vi "First Order System Demo.vi"() -> ()   [LabVIEW 2021]
panel:
  in  "Stop Button":bool
  out "First Order System Step Response":waveform(dbl)[](graph)
  in  "Final Value":dbl=1.0
  in  "Initial Value":dbl
  in  "Time constant [s]":dbl(slide)=1.0 scale=0.0..10.0
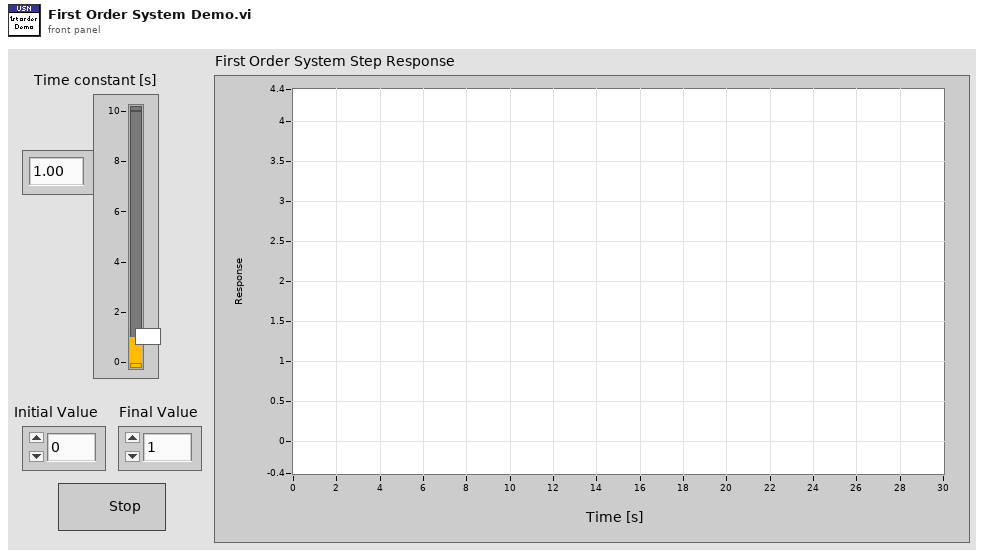
[diagram p1: front panel]
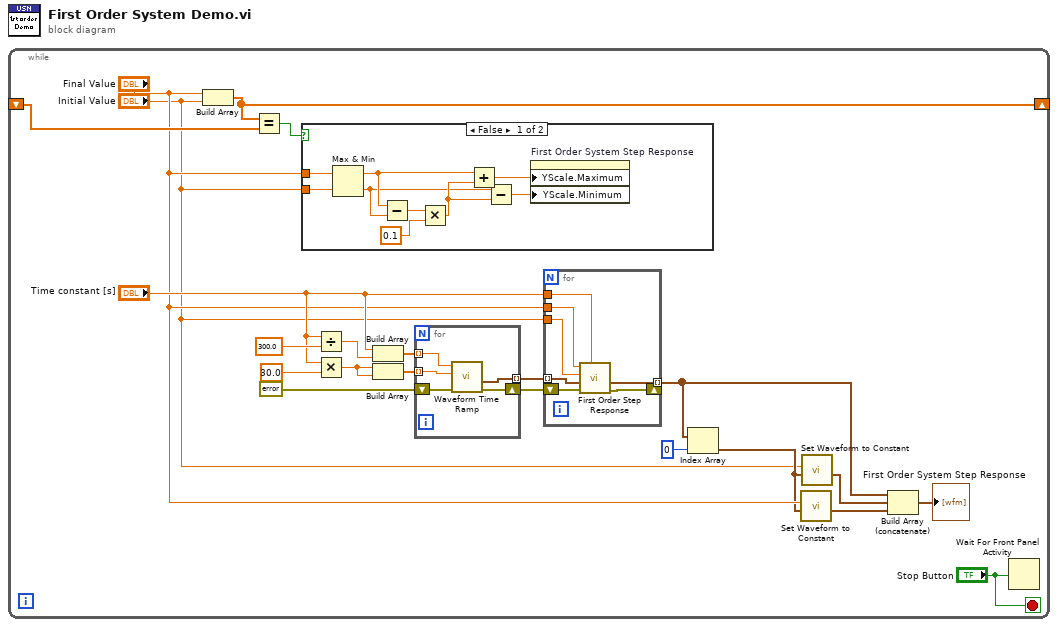
[diagram p0: block diagram]
diagram:
  n1 = while {
    shift-right: [w14] -> _
    shift-left: _ -> [w20]
    stop <- "Stop Button" stop-if-true
    n2 = Build Array("Final Value", "Initial Value") -> (w14:dbl[])
    n3 = Equal?(x=w14, y=w20) -> (x = y?=w19:bool)
    n4 = case shown="False" w19 {
      tunnel: "Final Value" -> [w29 _]
      tunnel: "Initial Value" -> [w28 _]
      frame False {
        n5 = Max & Min(x=w29, y=w28) -> (max(x,y)=w33:dbl, min(x,y)=w32:dbl)
        n6 = Subtract(x=w33, y=w32) -> (x-y=w36:dbl)
        n7 = Multiply(x=w36, y=0.1) -> (x*y=w34:dbl)
        n8 = Add(x=w33, y=w34) -> (x+y=w31:dbl)
        n9 = Subtract(x=w32, y=w34) -> (x-y=w30:dbl)
        n10 = property on="First Order System Step Response" class="WFGraph (strict)"("YScale.Maximum"=w31, "YScale.Minimum"=w30) -> ()  [unwired: 2 in, 2 out]
      }
      frame True {
      }
    }
    n11 = Divide(x="Time constant [s]", y=300.0) -> (x/y=w15:dbl)
    n12 = Multiply(x="Time constant [s]", y=30.0 ("x")) -> (x*y=w12:dbl)
    n13 = Build Array("Time constant [s]", w15) -> (w17:dbl[])
    n14 = Build Array(w12, w12) -> (w16:dbl[])
    n15 = for {
      tunnel: [w27] -> w11 mode=indexing
      tunnel: w17 -> [w26] mode=indexing
      tunnel: w16 -> [w25] mode=indexing
      shift-right: [w24] -> w2
      shift-left: errorcluster {"status"=FALSE, "code"=0, "source"=""} ("Error Out") -> [w23]
      n16 = call "Waveform Time Ramp.vi"("Error In"=w23, "End [s]"=w25, "dt [s]"=w26) -> ("Error Out"=w24:errorcluster, "Waveform Time Ramp"=w27:waveform(dbl))  [unwired: 7 in]
    }
    n17 = for {
      tunnel: "Initial Value" -> [w43]
      tunnel: "Final Value" -> [w42]
      tunnel: [w41] -> w9 mode=indexing
      tunnel: w11 -> [w39] mode=indexing
      tunnel: "Time constant [s]" -> [w40]
      shift-right: [w38] -> _
      shift-left: w2 -> [w37]
      n18 = call "First Order Step Response.vi"("Time constant [s]"=w40, "Error In"=w37, "Time Vector [s]"=w39, "Initial Value"=w43, "Final Value"=w42) -> ("Error Out"=w38:errorcluster, "Response"=w41:waveform(dbl))  [unwired: 5 in]
    }
    n19 = Index Array(array=w9, index=0) -> (element=w5:waveform(dbl))
    n20 = call "Set Waveform to Constant.vi"("Original Waveform"=w5, "New Value"="Final Value") -> ("New Waveform"=w7:waveform(dbl))  [unwired: 8 in, 1 out]
    n21 = call "Set Waveform to Constant.vi"("Original Waveform"=w5, "New Value"="Initial Value") -> ("New Waveform"=w3:waveform(dbl))  [unwired: 8 in, 1 out]
    n22 = Build Array (concatenate)(w9, w3, w7) -> (→"First Order System Step Response":waveform(dbl)[])
    n23 = Wait For Front Panel Activity(3:"Stop Button") -> ()  [unwired: 2 in, 1 out]
  }
